vi "Connect.vi"(8 "error in":errorcluster, 11 "DB-MySQL in":refnum<class "DB-MySQL.lvclass">=refnum) -> (0 "error out":errorcluster, 3 "DB-MySQL out":refnum<class "DB-MySQL.lvclass">)   [LabVIEW 2020, in "hse-db-mysql.lvlib" / "DB-MySQL.lvclass"]
doc: "____\nHAMPEL SOFTWARE ENGINEERING v1.4.0 (2023-12-19 09:52)"
uses:
  DB-MySQL.lvclass
  C:/GitLab-Runner/builds/7NHnU7RQc/0/open-source/hse-db/Source/DB-Interface/DB-Interface.lvclass
  DB-Interface/DB-Interface.lvclass/DB-Interface.ctl
  DB-MySQL.lvclass/DB-MySQL.ctl
  DB-Interface/DB-Interface.lvclass
  <vilib>/Hampel Software Engineering/MySQLNetCom/MySQLNetCom.lvlib
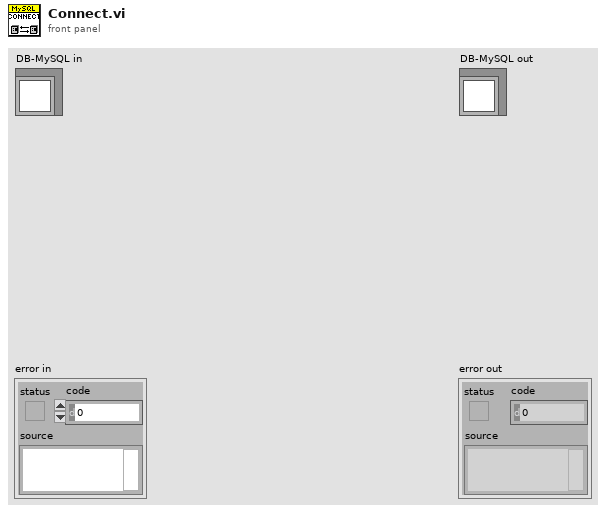
[diagram p1: front panel]
types:
  T1 = cluster{"User":string, "Password":string, "Database":string}
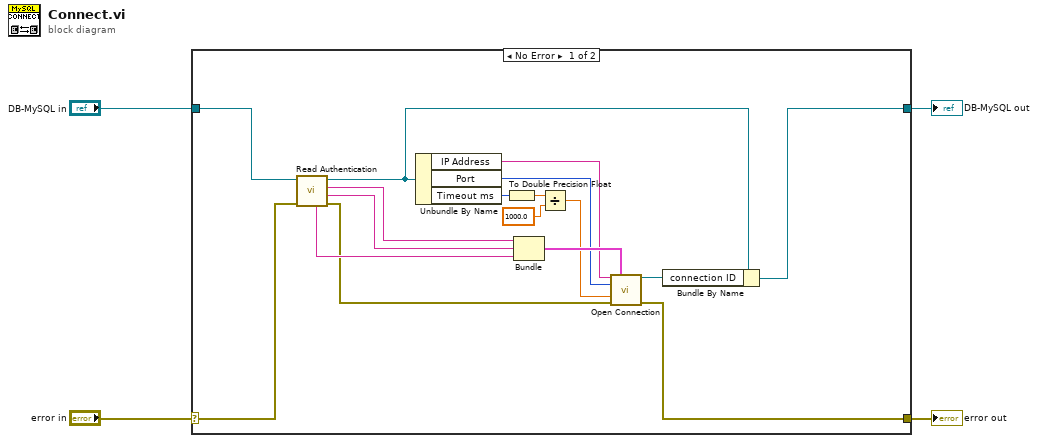
[diagram p0: block diagram]
diagram:
  n1 = case shown="No Error" "error in" {
    selector: "error in" -> [w21 w23]
    tunnel: [w10 w23] -> w3
    tunnel: [w12 w22] -> w1
    tunnel: "DB-MySQL in" -> [w20 w22]
    frame No Error {
      n2 = call "Read Authentication.vi"("error in"=w21, "DB-Engine in"=w20) -> ("error out"=w11:errorcluster, "Password"=w14:string, "User"=w15:string, "DB-Engine out"=w19:refnum<class "DB-MySQL.lvclass">, "Database"=w13:string)  [unwired: 5 in]
      n3 = Unbundle By Name(w19) -> ("IP Address"=w7:string, "Port"=w6:u16, "Timeout ms"=w18:i32)
      n4 = To Double Precision Float(number=w18) -> (double precision float=w17:dbl)
      n5 = Bundle("User"=w15, "Password"=w14, "Database"=w13) -> (w8:T1)  [unwired: 1 in]
      n6 = Divide(x=w17, y=1000.0) -> (x/y=w5:dbl)
      n7 = call <vilib>:"Open Connection.vi"("Server Address"=w7, "Authentication"=w8, "Port (3306)"=w6, "timeout (15s)"=w5, "error in (no error)"=w11) -> ("connection ID out"=w9:refnum<k5>, "error out"=w10:errorcluster)  [unwired: 9 in]
      n8 = Bundle By Name(cluster=w19, "connection ID"=w9) -> (w12:refnum<class "DB-MySQL.lvclass">)
    }
    frame Error {
    }
  }
  "error out" <- w3
  "DB-MySQL out" <- w1
